vi "Script Test Utility.vi"() -> ()   [LabVIEW 2013]
uses:
  <instrlib>/niHSDIO/niHSDIO.llb/niHSDIO_ctl Trigger Script - trigID Values (Ring).ctl
  <instrlib>/niHSDIO/niHSDIO.llb/niHSDIO_ctl Generation Mode Values (Ring).ctl
  <instrlib>/niHSDIO/niHSDIO.llb/niHSDIO_ctl Exported Signal Desination Values (ComboBox).ctl
  <instrlib>/niHSDIO/niHSDIO.llb/niHSDIO_ctl Exported Signal Name Values (Ring).ctl
  <instrlib>/niHSDIO/niHSDIO.llb/niHSDIO_ctl Data Position Values (Ring).ctl
  <instrlib>/niHSDIO/niHSDIO.llb/niHSDIO Configure Software Script Trigger.vi
  <instrlib>/niHSDIO/niHSDIO.llb/niHSDIO Configure Data Voltage Custom Levels.vi
  <instrlib>/niHSDIO/niHSDIO.llb/niHSDIO Configure Initial State (String).vi
  <instrlib>/niHSDIO/niHSDIO.llb/niHSDIO Configure Idle State (String).vi
  <instrlib>/niHSDIO/niHSDIO.llb/niHSDIO Write Named Waveform From File (HWS).vi
  <instrlib>/niHSDIO/niHSDIO.llb/niHSDIO_ctl Trigger SW - TrigName Values (Ring).ctl
panel:
  in  "Script Steps":string="generate HV29"
  in  "Script Name":string="test"
  in  "channel list (all:\"\") 2":string="2,0,6"
  in  "Resource name":refnum<k15>="6556"
  in  "Clock Rate":dbl=50000000.0 format="%.2p"
  in  "high level (3.30 volts)":dbl=1.8 format="%.2f"
  in  "low level (0.00 volts)":dbl format="%.2f"
  in  "Application Directory":path=path "C:/Users/user/Documents/AD2240/Waveforms/RFFE6"
  # "generate ActiveMode\n generate UnlockQ\n generate UnlockR\n generate UnlockV\n generate HV13"
  # "LowPowerMode"
  # "Generate State00\n\tGenerate State15\n\t Generate SWReset"
  # "// Date: 9/21/2022 11:41:04 AM\n// Chipset: Switch_RFFE\n// Family: AD2240_0.1  LoaderVersion:7.15.2.0\n// Frequency: 1,000,000 Hz\nDELAY 00000014  //Delay in usec\n1C  00B8  // Reg28\nDELAY 00004E20  //Delay in usec\n1C  0038  // Reg28\nREAD_REG 1C  //Read Register\n1F  0051  // Reg31\n1F  0052  // Reg31\n1F  0056  // Reg31\n41  005D  // Reg65\nREAD_REG 5D  //Read Register\n41  005C  // Reg65\nREAD_REG 5C  //Read Register\n41  0050  // Reg65\nREAD_REG 50  //Read Register"
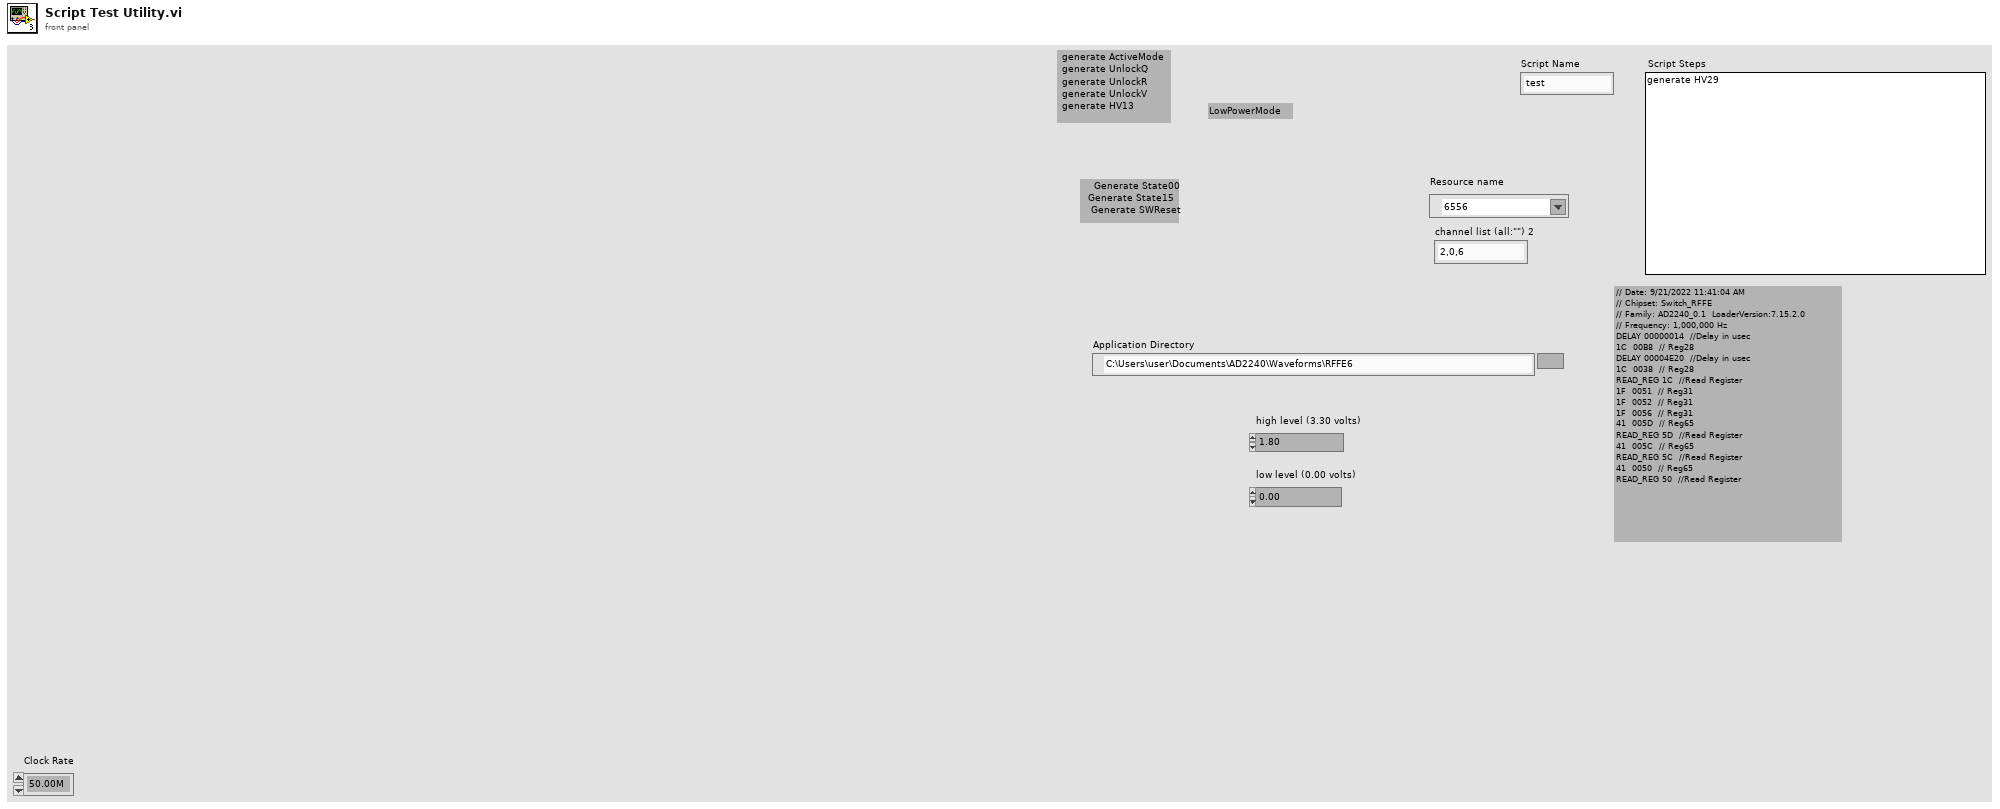
[diagram p1: front panel]
types:
  T1 = typedef "niHSDIO_ctl Data Position Values (Ring).ctl" = i32
  T2 = typedef "niHSDIO_ctl Exported Signal Name Values (Ring).ctl" = u16
  T3 = typedef "niHSDIO_ctl Exported Signal Desination Values (ComboBox).ctl" = string
  T4 = typedef "niHSDIO_ctl Generation Mode Values (Ring).ctl" = i32
  T5 = typedef "niHSDIO_ctl Trigger Script - trigID Values (Ring).ctl" = string
  T6 = typedef "niHSDIO_ctl Trigger SW - TrigName Values (Ring).ctl" = i32
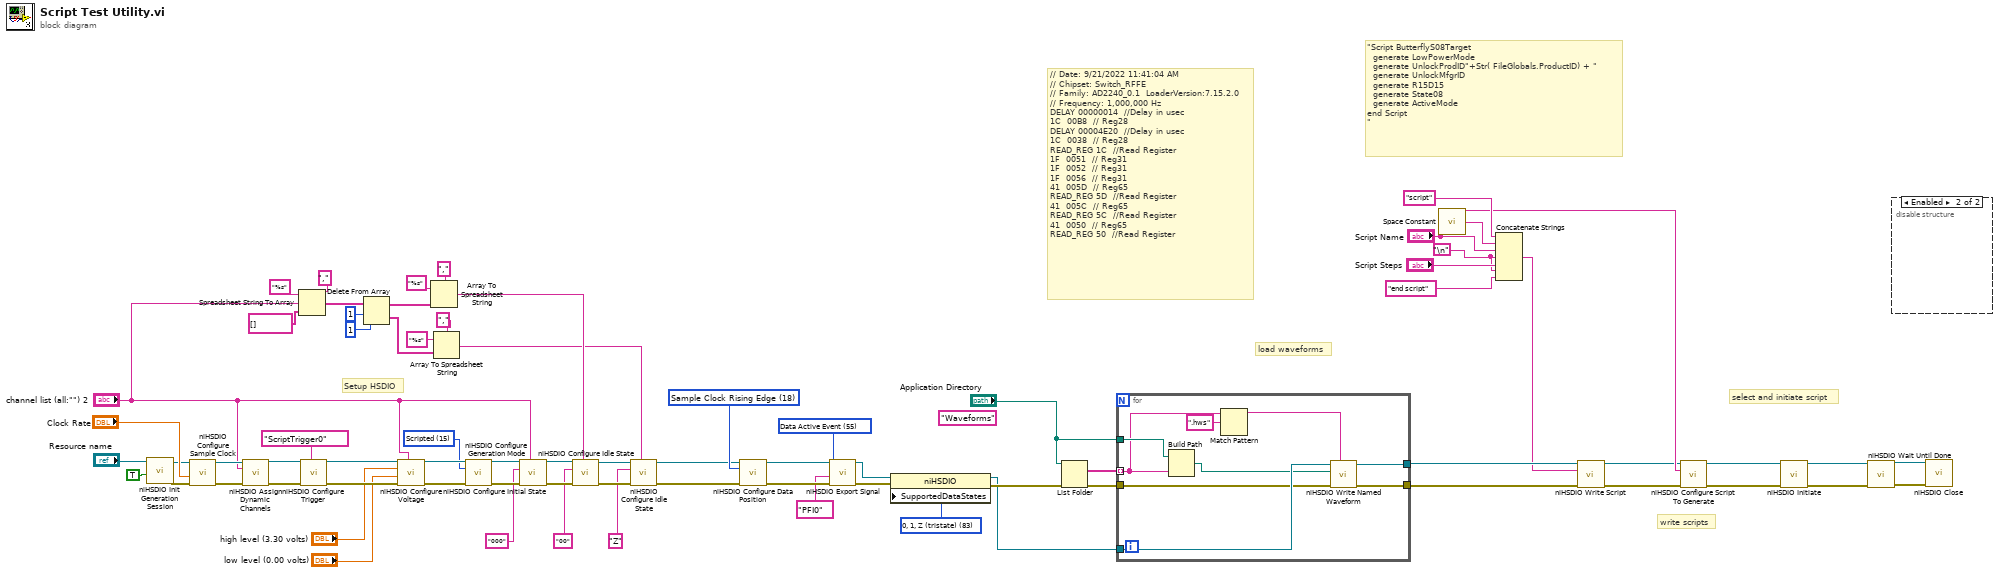
[diagram p0: block diagram]
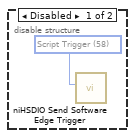
[diagram p2: hidden frame]
diagram:
  w25 = "\n"
  w51 = T1 18 items=["Sample Clock Rising Edge"=18, "Sample Clock Falling Edge"=19, "Delay from Sample Clock Rising Edge"=20] ("position (rising edge)")
  w57 = T2 55 items=["Sample Clock"=51, "Reference Clock"=52, "Start Trigger"=53, "Reference Trigger"=54, "Advance Trigger"=61, "Pause Trigger"=57, "Script Trigger"=58, "Stop Trigger"=82, "Data Active Event"=55, "Marker Event"=59, "Ready For Start Event"=56, "Ready For Advance Event"=66, "End Of Record Event"=68, "Onboard Ref Clock"=60] ("signal (sample clock)")
  w58 = 83 items=["0, 1 (binary)"=77, "0, 1, Z (tristate)"=83, "0, 1, Z, L, H, X (stim/resp)"=78, "L, H, X (resp only)"=79] ("Advanced:Supported Data States")
  w65 = T4 15 items=["Waveform"=14, "Scripted"=15] ("generation mode (waveform)")
  (unwired) "Waveforms" ("string")
  # "// Date: 9/21/2022 11:41:04 AM\n// Chipset: Switch_RFFE\n// Family: AD2240_0.1  LoaderVersion:7.15.2.0\n// Frequency: 1,000,000 Hz\nDELAY 00000014  //Delay in usec\n1C  00B8  // Reg28\nDELAY 00004E20  //Delay in usec\n1C  0038  // Reg28\nREAD_REG 1C  //Read Register\n1F  0051  // Reg31\n1F  0052  // Reg31\n1F  0056  // Reg31\n41  005D  // Reg65\nREAD_REG 5D  //Read Register\n41  005C  // Reg65\nREAD_REG 5C  //Read Register\n41  0050  // Reg65\nREAD_REG 50  //Read Register"
  # "\"Script ButterflyS08Target\n  generate LowPowerMode\n  generate UnlockProdID\"+Str( FileGlobals.ProductID) + \"\n  generate UnlockMfgrID\n  generate R15D15\n  generate State08\n  generate ActiveMode\nend Script\n\""
  # "select and initiate script"
  # "write scripts"
  # "load waveforms"
  # "Setup HSDIO"
  n1 = call <instrlib>:"niHSDIO Init Generation Session.vi"("reset instrument (no:F)"=TRUE, "resource name"="Resource name") -> ("error out"=w50:errorcluster, "instrument handle out"=w47:refnum<k15>)  [unwired: 8 in]
  n2 = call <instrlib>:"niHSDIO Configure Sample Clock.vi"("error in (no error)"=w50, "clock rate (50MHz)"="Clock Rate", "instrument handle"=w47) -> ("error out"=w49:errorcluster, "instrument handle out"=w48:refnum<k15>)  [unwired: 7 in]
  n3 = call <instrlib>:"niHSDIO Assign Dynamic Channels.vi"("error in (no error)"=w49, "channel list (all:\"\")"="channel list (all:\"\") 2", "instrument handle"=w48) -> ("error out"=w72:errorcluster, "instrument handle out"=w71:refnum<k15>)  [unwired: 7 in]
  n4 = Spreadsheet String To Array(delimiter (Tab)=",", format string="%s", spreadsheet string="channel list (all:\"\") 2", array type (2D Dbl)=string[] []) -> (array=w20:string[])
  n5 = call-poly <instrlib>:"niHSDIO Configure Trigger.vi"("trigger id (script trigger 0)"=T5 "ScriptTrigger0", "error in (no error)"=w72, "instrument handle"=w71) -> ("error out"=w69:errorcluster, "instrument handle out"=w68:refnum<k15>)  [unwired: 7 in]
  n6 = Delete From Array(array=w20, length=1, index=1) -> (deleted portion=w16:string[], array with subset deleted=w17:string[])
  n7 = call-poly <instrlib>:"niHSDIO Configure Voltage.vi"("channel list (all:\"\")"="channel list (all:\"\") 2", "error in (no error)"=w69, "low level (0.00 volts)"="low level (0.00 volts)", "high level (3.30 volts)"="high level (3.30 volts)", "instrument handle"=w68) -> ("error out"=w67:errorcluster, "instrument handle out"=w66:refnum<k15>)  [unwired: 5 in]
  n8 = Array To Spreadsheet String(delimiter (Tab)=",", array=w17, 3:"%s" ("format string")) -> (spreadsheet string=w3:string)
  n9 = Array To Spreadsheet String(delimiter (Tab)=",", array=w16, 3:"%s" ("format string")) -> (spreadsheet string=w1:string)
  n10 = call <instrlib>:"niHSDIO Configure Generation Mode.vi"("error in (no error)"=w67, "generation mode (waveform)"=w65, "instrument handle"=w66) -> ("error out"=w64:errorcluster, "instrument handle out"=w61:refnum<k15>)  [unwired: 7 in]
  n11 = call-poly <instrlib>:"niHSDIO Configure Initial State.vi"("channel list"="channel list (all:\"\") 2", "error in (no error)"=w64, "initial state"="000" ("idle state"), "instrument handle"=w61) -> ("error out"=w63:errorcluster, "instrument handle out"=w62:refnum<k15>)  [unwired: 6 in]
  n12 = call-poly <instrlib>:"niHSDIO Configure Idle State.vi"("channel list"=w3, "error in (no error)"=w63, "idle state"="00", "instrument handle"=w62) -> ("error out"=w10:errorcluster, "instrument handle out"=w7:refnum<k15>)  [unwired: 6 in]
  n13 = call-poly <instrlib>:"niHSDIO Configure Idle State.vi"("channel list"=w1, "error in (no error)"=w10, "idle state"="Z", "instrument handle"=w7) -> ("error out"=w9:errorcluster, "instrument handle out"=w8:refnum<k15>)  [unwired: 6 in]
  n14 = call <instrlib>:"niHSDIO Configure Data Position.vi"("error in (no error)"=w9, "position (rising edge)"=w51, "instrument handle"=w8) -> ("error out"=w56:errorcluster, "instrument handle out"=w55:refnum<k15>)  [unwired: 7 in]
  n15 = call <instrlib>:"niHSDIO Export Signal.vi"("error in (no error)"=w56, "output terminal (do not export)"=T3 "PFI0", "signal (sample clock)"=w57, "instrument handle"=w55) -> ("error out"=w53:errorcluster, "instrument handle out"=w52:refnum<k15>)  [unwired: 6 in]
  n16 = property on="Property Node" class="niHSDIO"(reference=w52, error in=w53, "SupportedDataStates"=w58) -> (reference out=w26:refnum<k15>, error out=w46:errorcluster)
  n17 = List Folder(path="Application Directory", error in=w46) -> (filenames=w30:string[], error out=w28:errorcluster)  [unwired: 2 in, 2 out]
  n18 = for {
    tunnel: [w82] -> w43
    tunnel: [w81] -> w39
    tunnel: w26 -> [w80]
    tunnel: w30 -> [w76] mode=indexing
    tunnel: "Application Directory" -> [w78]
    tunnel: w28 -> [w79]
    n19 = Build Path(base path=w78, name or relative path=w76) -> (appended path=w77:path)
    n20 = Match Pattern(string=w76, regular expression=".hws") -> (before substring=w74:string)  [unwired: 1 in, 3 out]
    n21 = call-poly <instrlib>:"niHSDIO Write Named Waveform.vi"("waveform name (default:\"\")"=w74, "error in (no error)"=w79, "file path"=w77, "instrument handle"=w80) -> ("error out"=w82:errorcluster, "instrument handle out"=w81:refnum<k15>)  [unwired: 5 in, 1 out]
  }
  n22 = call <vilib>:"Space Constant.vi"() -> ("String"=w44:string)
  n23 = Concatenate Strings("script" ("string"), w44, "Script Name", w25, "Script Steps", w25, "end script") -> (w38:string)
  n24 = call <instrlib>:"niHSDIO Write Script.vi"("error in (no error)"=w43, "script"=w38, "instrument handle"=w39) -> ("error out"=w42:errorcluster, "instrument handle out"=w40:refnum<k15>)  [unwired: 7 in]
  n25 = call <instrlib>:"niHSDIO Configure Script To Generate.vi"("error in (no error)"=w42, "script name"="Script Name", "instrument handle"=w40) -> ("error out"=w36:errorcluster, "instrument handle out"=w35:refnum<k15>)  [unwired: 7 in]
  n26 = call <instrlib>:"niHSDIO Initiate.vi"("error in (no error)"=w36, "instrument handle"=w35) -> ("error out"=w34:errorcluster, "instrument handle out"=w33:refnum<k15>)  [unwired: 8 in]
  n27 = call <instrlib>:"niHSDIO Wait Until Done.vi"("error in (no error)"=w34, "instrument handle"=w33) -> ("error out"=w32:errorcluster, "instrument handle out"=w31:refnum<k15>)  [unwired: 8 in]
  n28 = disable-structure shown="Enabled" {
    frame Disabled {
      w83 = T6 58 items=["Start Trigger"=53, "Reference Trigger"=54, "Advance Trigger"=61, "Script Trigger"=58, "Stop Trigger"=82] ("trigger (start trigger)")
      n29 = call <instrlib>:"niHSDIO Send Software Edge Trigger.vi"("trigger (start trigger)"=w83) -> ()  [unwired: 9 in, 2 out]
    }
    frame Enabled {
    }
  }
  n30 = call <instrlib>:"niHSDIO Close.vi"("error in (no error)"=w32, "instrument handle"=w31) -> ()  [unwired: 9 in, 1 out]
